vi "Get Start Delay.vi"() -> (2 "Encoder out":i32, 3 "Start Delay(in)":sgl)   [LabVIEW 2015, in "Tool Cfg.lvlib"]
uses:
  Tool Cfg.lvlib
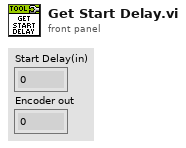
[diagram p1: front panel]
types:
  T1 = typedef "Tool Cfg.lvlib/_Tool Block Cluster_v3--typedef.ctl" = cluster{"Encoder Size":u16, "Encoder Scale":u32, "Encoder Offset":i32, "MaxEncoder":i32, "MinEncoder":i32, "Start Delay":sgl, "Tool Face Ref":sgl}
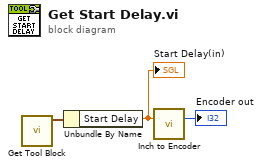
[diagram p0: block diagram]
diagram:
  n1 = call "Get Tool Block.vi"() -> ("Tool Block"=w3:T1)  [unwired: 11 in]
  n2 = Unbundle By Name(w3) -> ("Start Delay"=w2:sgl)
  "Start Delay(in)" <- w2
  n3 = call "Inch to Encoder.vi"("Inches in"=w2) -> ("Encoder out"=→"Encoder out":i32)  [unwired: 14 in]
